vi "SN_validator.vi"(6 "Length range":T3, 7 "Validaton mode":T5, 8 "error in (no error)":errorcluster, 9 "SN Regex":string[][](array[string]), 10 "Device Type":T4, 11 "SN in":string) -> (0 "error out":errorcluster, 3 "SN Data":T1)   [LabVIEW 2024, in "SN Validator.lvlib"]
doc: "Modular Serial Number Parser for Internal Device Validation — A configurable LabVIEW subVI designed to validate serial numbers based on format, length, and device type (BGH Product, BGH Asset, Samsung Product). Supports multiple parsing modes and external regex configuration for flexible integration in production test systems."
uses:
  SN Validator.lvlib
  <vilib>/ErrorRing/Error Ring.xnode
  SN_device_type_out.ctl
  SN Data.ctl
  SN_device_type.ctl
  SN_length.ctl
  SN_validation_mode.ctl
  <vilib>/TABOADA/Event-Driven Queued SM/Event-Driven QSM/ED Queued State Machine.lvlib
  <vilib>/TABOADA/Event-Driven Queued SM/Event-Driven QSM/queue state & data (Array).vi
  data--cluster.ctl
  <vilib>/Utility/error.llb/Error Cluster From Error Code.vi
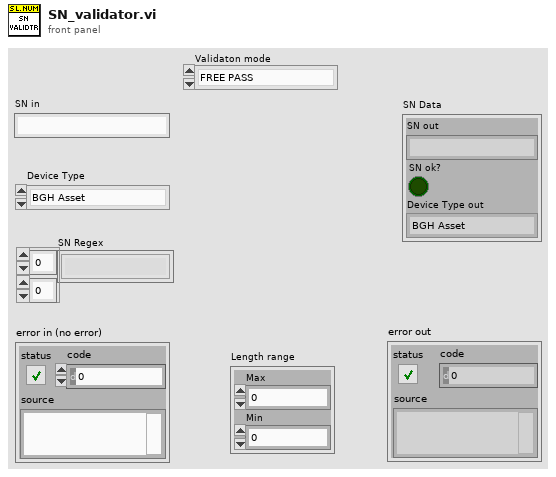
[diagram p1: front panel]
types:
  T1 = typedef "SN Validator.lvlib/SN Data.ctl" = cluster{"SN out":string, "SN ok?":bool, "Device Type out":T2}
  T2 = typedef "SN Validator.lvlib/SN_device_type_out.ctl" = enum16{"BGH Asset", "BGH Product", "SAMSUNG Product", "GENERIC Product", "No Product", ""}
  T3 = typedef "SN Validator.lvlib/SN_length.ctl" = cluster{"Max":i32, "Min":i32}
  T4 = typedef "SN Validator.lvlib/SN_device_type.ctl" = enum16{"BGH Asset", "BGH Product", "SAMSUNG Product"}
  T5 = typedef "SN Validator.lvlib/SN_validation_mode.ctl" = enum16{"FREE PASS", "LENGTH BASED", "REGEX BASED", "AUTO"}
  T6 = typedef "SN Validator.lvlib/data--cluster.ctl" = cluster{"Serial Number":string, "SN ok?":bool, "SN Regex":string[][], "Validaton mode":T5, "Length range":T3, "Device Type":T4, "Device Type out":T2}
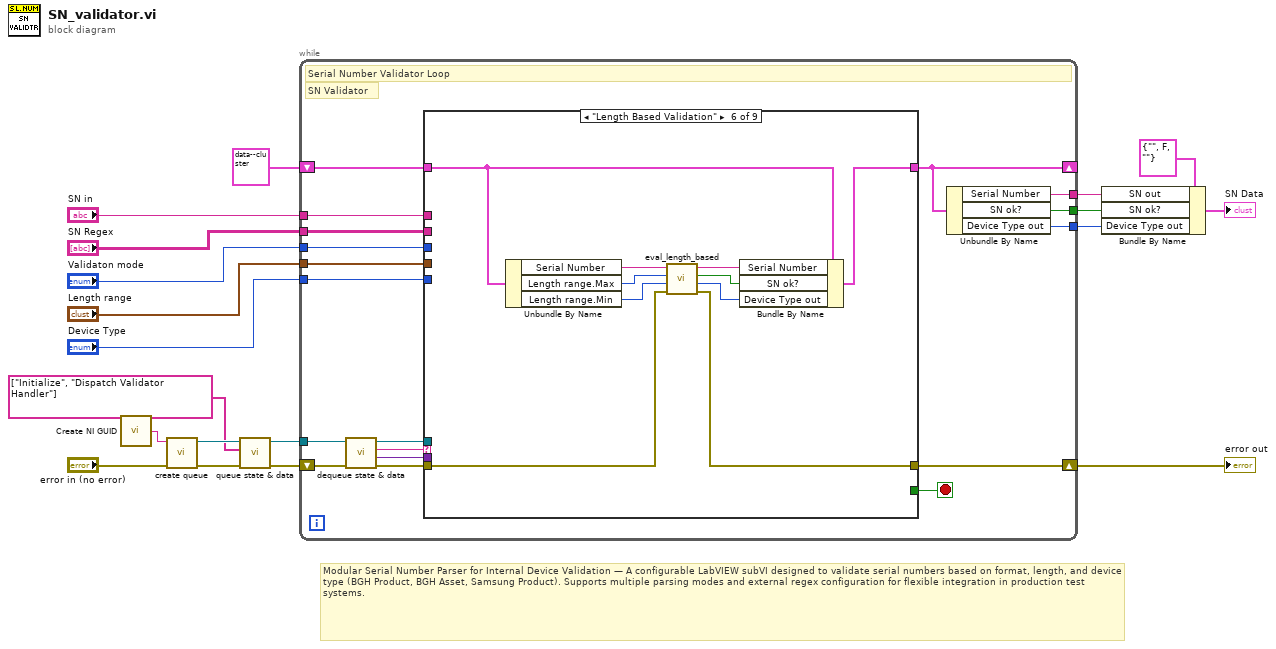
[diagram p0: block diagram]
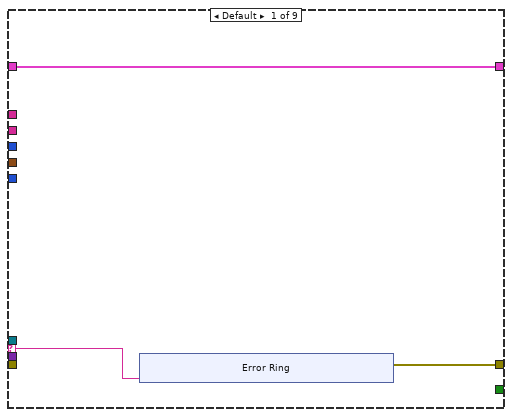
[diagram p2: hidden frame]
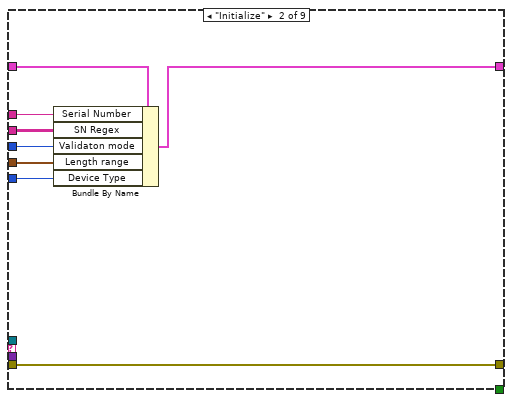
[diagram p3: hidden frame]
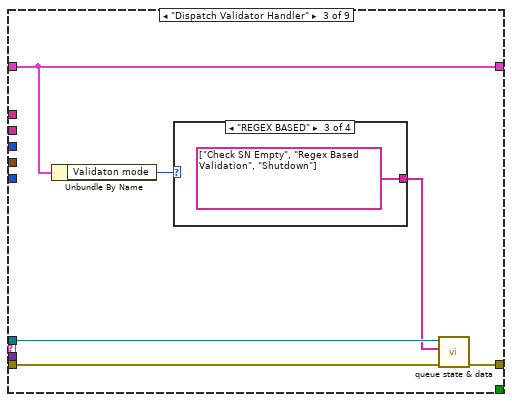
[diagram p4: hidden frame]
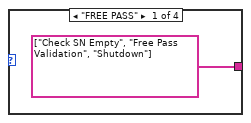
[diagram p5: hidden frame]
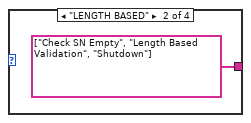
[diagram p6: hidden frame]
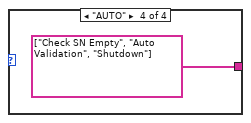
[diagram p7: hidden frame]
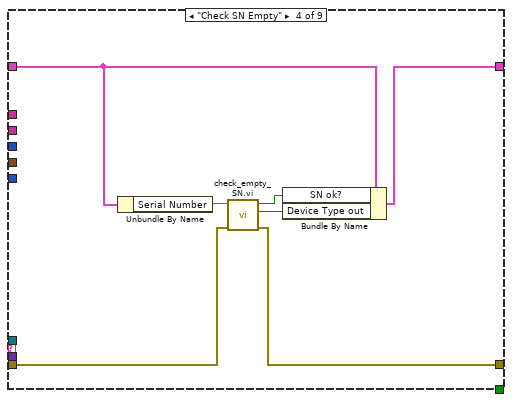
[diagram p8: hidden frame]
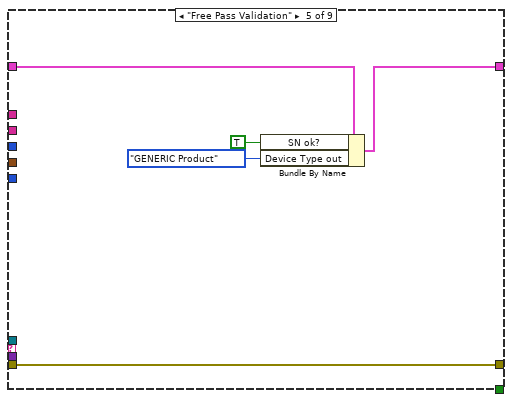
[diagram p9: hidden frame]
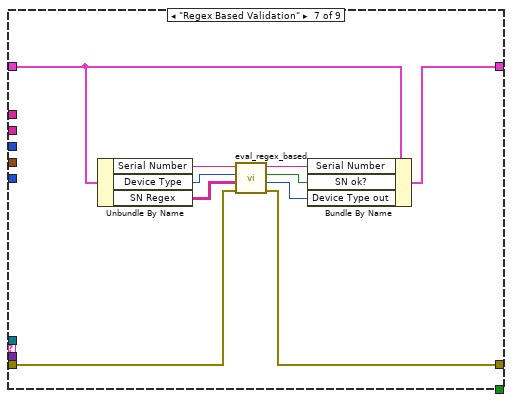
[diagram p10: hidden frame]
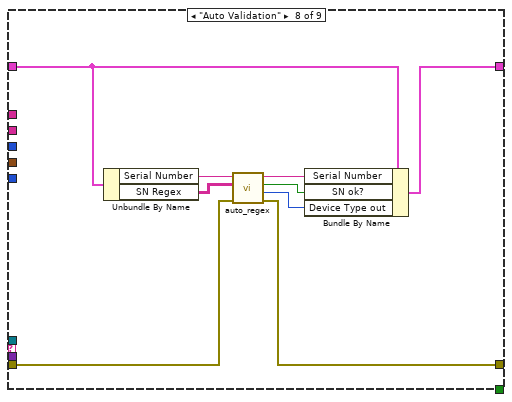
[diagram p11: hidden frame]
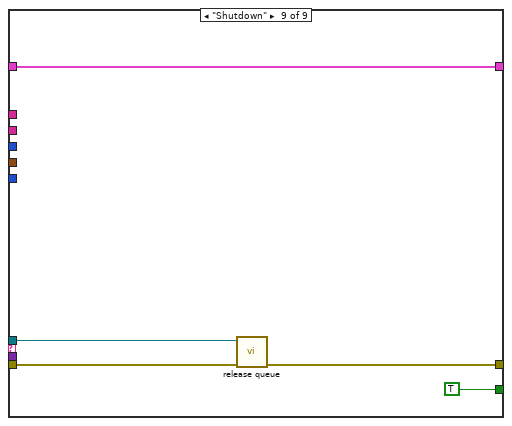
[diagram p12: hidden frame]
diagram:
  # "Modular Serial Number Parser for Internal Device Validation — A configurable LabVIEW subVI designed to validate serial numbers based on format, length, and device type (BGH Product, BGH Asset, Samsung Product). Supports multiple parsing modes and external regex configuration for flexible integration in production test systems."
  n1 = call <vilib>:"Create NI GUID.vi"() -> ("NI GUID"=w2:string)
  n2 = call <vilib>:"create queue.vi"("error in (no error)"="error in (no error)", "name (unnamed)"=w2) -> ("error out"=w6:errorcluster, "queue out"=w7:refnum<queue>)  [unwired: 7 in, 1 out]
  n3 = call-poly <vilib>:"queue state & data.vi"("error in (no error)"=w6, "State Array"=string[] ["Initialize", "Dispatch Validator Handler"], "queue in"=w7) -> ("error out"=w5:errorcluster, "queue out"=w3:refnum<queue>)  [unwired: 7 in]
  n4 = while {
    shift-right: [w30] -> w15
    shift-left: w5 -> [w25]
    tunnel: w3 -> [w24]
    shift-right: [w26] -> _
    shift-left: T6 {"Serial Number"="", "SN ok?"=FALSE, "SN Regex"=[], "Validaton mode"=enum."FREE PASS", "Length range"={"Max"=0, "Min"=0}, "Device Type"=enum."BGH Asset", "Device Type out"=enum."BGH Asset"} ("Data") -> [w36]
    tunnel: "SN in" -> [w35]
    tunnel: "SN Regex" -> [w34]
    tunnel: "Validaton mode" -> [w33]
    tunnel: "Length range" -> [w32]
    tunnel: "Device Type" -> [w31]
    tunnel: [w29] -> w11
    tunnel: [w28] -> w10
    tunnel: [w27] -> w9
    stop <- w37 stop-if-true
    # "SN Validator"
    # "Serial Number Validator Loop"
    n5 = call <vilib>:"dequeue state & data.vi"("error in (no error)"=w25, "queue in"=w24) -> ("error out"=w20:errorcluster, "State Data"=w21:variant, "State"=w22:string, "queue out"=w23:refnum<queue>)  [unwired: 6 in]
    n6 = case shown="\"Length Based Validation\"" w22 {
      selector: w22 -> [w39 _ _ _ _ _ _ _ _]
      tunnel: w20 -> [_ w48 w58 w69 w73 w87 w89 w100 w108]
      tunnel: [w38 w48 w59 w66 w73 w78 w88 w98 w107] -> w30
      tunnel: [_ _ _ _ _ _ _ _ TRUE] -> w37
      tunnel: w23 -> [_ _ w57 _ _ _ _ _ w109]
      tunnel: w21 -> [_ _ _ _ _ _ _ _ _]
      tunnel: w36 -> [w40 w55 w61 w72 w77 w83 w95 w104 w110]
      tunnel: [w40 w54 w61 w71 w76 w82 w94 w103 w110] -> w26
      tunnel: w35 -> [_ w53 _ _ _ _ _ _ _]
      tunnel: w34 -> [_ w52 _ _ _ _ _ _ _]
      tunnel: w33 -> [_ w50 _ _ _ _ _ _ _]
      tunnel: w32 -> [_ w51 _ _ _ _ _ _ _]
      tunnel: w31 -> [_ w49 _ _ _ _ _ _ _]
      frame Default {
        n7 = xnode ("Error Ring")("parameter 0"=w39) -> ("error out"=w38:errorcluster)
      }
      frame "Initialize" {
        n8 = Bundle By Name(cluster=w55, "Serial Number"=w53, "SN Regex"=w52, "Validaton mode"=w50, "Length range"=w51, "Device Type"=w49) -> (w54:T6)
      }
      frame "Dispatch Validator Handler" {
        n9 = Unbundle By Name(w61) -> ("Validaton mode"=w60:T5)
        n10 = case shown="\"REGEX BASED\"" w60 {
          tunnel: [string[] ["Check SN Empty", "Free Pass Validation", "Shutdown"] string[] ["Check SN Empty", "Length Based Validation", "Shutdown"] string[] ["Check SN Empty", "Regex Based Validation", "Shutdown"] string[] ["Check SN Empty", "Auto Validation", "Shutdown"]] -> w56
          frame "FREE PASS" {
          }
          frame "LENGTH BASED" {
          }
          frame "REGEX BASED" {
          }
          frame "AUTO" {
          }
        }
        n11 = call-poly <vilib>:"queue state & data.vi"("error in (no error)"=w58, "State Array"=w56, "queue in"=w57) -> ("error out"=w59:errorcluster)  [unwired: 7 in, 1 out]
      }
      frame "Check SN Empty" {
        n12 = Unbundle By Name(w72) -> ("Serial Number"=w68:string)
        n13 = call "check_empty_SN.vi.vi"("error in (no error)"=w69, "SN"=w68) -> ("error out"=w66:errorcluster, "Device Type out"=w67:T2, "SN ok?"=w70:bool)  [unwired: 7 in]
        n14 = Bundle By Name(cluster=w72, "SN ok?"=w70, "Device Type out"=w67) -> (w71:T6)
      }
      frame "Free Pass Validation" {
        n15 = Bundle By Name(cluster=w77, "SN ok?"=TRUE, "Device Type out"=SN_device_type_out."GENERIC Product") -> (w76:T6)
      }
      frame "Length Based Validation" {
        n16 = Unbundle By Name(w83) -> ("Serial Number"=w84:string, "Length range.Max"=w86:i32, "Length range.Min"=w85:i32)
        n17 = call "eval_length_based.vi"("error in (no error)"=w87, "Min"=w85, "Max"=w86, "SN"=w84) -> ("error out"=w78:errorcluster, "Device Type out"=w79:T2, "SN ok?"=w80:bool, "SN out"=w81:string)  [unwired: 4 in]
        n18 = Bundle By Name(cluster=w83, "Serial Number"=w81, "SN ok?"=w80, "Device Type out"=w79) -> (w82:T6)
      }
      frame "Regex Based Validation" {
        n19 = Unbundle By Name(w95) -> ("Serial Number"=w97:string, "Device Type"=w96:T4, "SN Regex"=w93:string[][])
        n20 = call "eval_regex_based.vi"("error in (no error)"=w89, "Regex"=w93, "Device Type"=w96, "SN"=w97) -> ("error out"=w88:errorcluster, "Device Type out"=w92:T2, "SN ok?"=w91:bool, "SN out"=w90:string)  [unwired: 4 in]
        n21 = Bundle By Name(cluster=w95, "Serial Number"=w90, "SN ok?"=w91, "Device Type out"=w92) -> (w94:T6)
      }
      frame "Auto Validation" {
        n22 = Unbundle By Name(w104) -> ("Serial Number"=w106:string, "SN Regex"=w105:string[][])
        n23 = call "auto_regex.vi"("error in (no error)"=w100, "Regex"=w105, "SN"=w106) -> ("error out"=w98:errorcluster, "Device Type out"=w101:T2, "SN ok?"=w99:bool, "SN out"=w102:string)  [unwired: 5 in]
        n24 = Bundle By Name(cluster=w104, "Serial Number"=w102, "SN ok?"=w99, "Device Type out"=w101) -> (w103:T6)
      }
      frame "Shutdown" {
        n25 = call <vilib>:"release queue.vi"("error in (no error)"=w108, "Queue in"=w109) -> ("error out"=w107:errorcluster)  [unwired: 9 in]
      }
    }
    n26 = Unbundle By Name(w26) -> ("Serial Number"=w29:string, "SN ok?"=w28:bool, "Device Type out"=w27:T2)
  }
  "error out" <- w15
  n27 = Bundle By Name(cluster=T1 {"SN out"="", "SN ok?"=FALSE, "Device Type out"=enum.""} ("SN Data"), "SN out"=w11, "SN ok?"=w10, "Device Type out"=w9) -> (→"SN Data":T1)
